vi "runtest build javascript enumeration array.vi"(1 "FIELD ID (\"\")":string, 2 "Enumerations":string[](array[string])) -> (0 "javascript Enumeration Array":string)   [LabVIEW 2011]
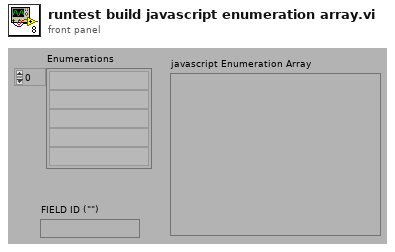
[diagram p1: front panel]
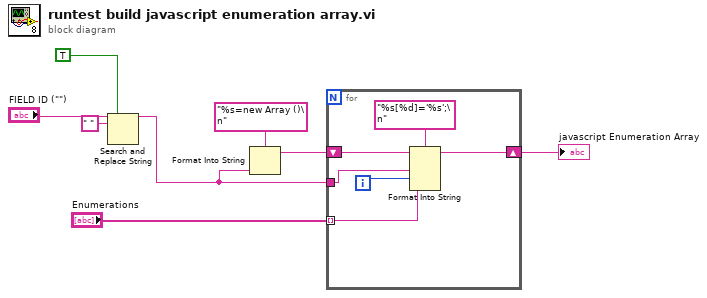
[diagram p0: block diagram]
diagram:
  n1 = Search and Replace String(replace all?=TRUE, input string="FIELD ID (\"\")", search string=" ") -> (result string=w1:string)  [unwired: 1 in, 7 out]
  n2 = Format Into String(format string="%s=new Array ()\n", w1) -> (resulting string=w7:string)  [unwired: 2 in, 1 out]
  n3 = for {
    shift-right: [w12] -> w5
    shift-left: w7 -> [w13]
    tunnel: "Enumerations" -> [w9] mode=indexing
    tunnel: w1 -> [w11]
    i -> [w10]
    n4 = Format Into String(format string="%s[%d]='%s';\n", initial string=w13, w11, w10, w9) -> (resulting string=w12:string)  [unwired: 1 in, 1 out]
  }
  "javascript Enumeration Array" <- w5
